vi "Strip VI Name.vi"(9 "Full VI Name":string="LMH-LINX.lvlib:ADXL345.lvlib:Close.vi") -> (2 "Path Tokens":string[](array[string]), 3 "Stripped Name":string)   [LabVIEW 2014]
doc: "Strips the namspacing (lvlibs) from the VI name.\n\nReturns lvlibs as path tokens, stripped to pretty names excluding top level lvlib.\ns"
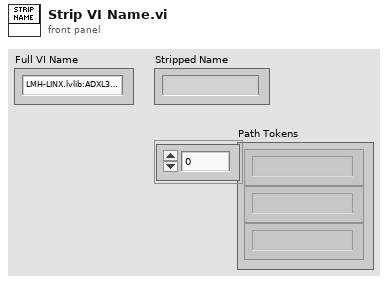
[diagram p1: front panel]
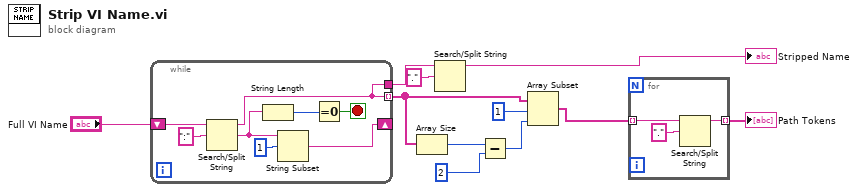
[diagram p0: block diagram]
diagram:
  n1 = while {
    shift-right: [w14] -> _
    shift-left: "Full VI Name" -> [w19]
    tunnel: [w12] -> w8
    tunnel: [w12] -> w6 mode=indexing
    stop <- w15 stop-if-true
    n2 = Search/Split String(string=w19, search string/char (-)=":") -> (substring before match=w12:string, match + rest of string=w13:string)  [unwired: 1 in, 1 out]
    n3 = String Length(string=w13) -> (length=w17:i32)
    n4 = String Subset(string=w13, offset (0)=1) -> (substring=w14:string)  [unwired: 1 in]
    n5 = Equal To 0?(x=w17) -> (x = 0?=w15:bool)
  }
  n6 = Array Size(array=w6) -> (size(s)=w2:i32)
  n7 = Search/Split String(string=w8, search string/char (-)=".") -> (substring before match=→"Stripped Name":string)  [unwired: 1 in, 2 out]
  n8 = Subtract(x=w2, y=2) -> (x-y=w3:i32)
  n9 = Array Subset(array=w6, index=1 ("length"), length=w3) -> (w5:string[])
  n10 = for {
    tunnel: w5 -> [w21] mode=indexing
    tunnel: [w20] -> w7 mode=indexing
    n11 = Search/Split String(string=w21, search string/char (-)=".") -> (substring before match=w20:string)  [unwired: 1 in, 2 out]
  }
  "Path Tokens" <- w7
